vi "PDSS - Add Error Message.vi"(8 "error in (no error)":errorcluster, 9 "is warning? (False)":bool=TRUE, 10 "error code (0)":i32=5005, 11 "error message (\"\")":string) -> (0 "error out":errorcluster, 3 "Current Message":string)   [LabVIEW 2014]
doc: "Use this template to build a VI to use as a subVI."
panel:
  in  "show call chain? (False)":bool
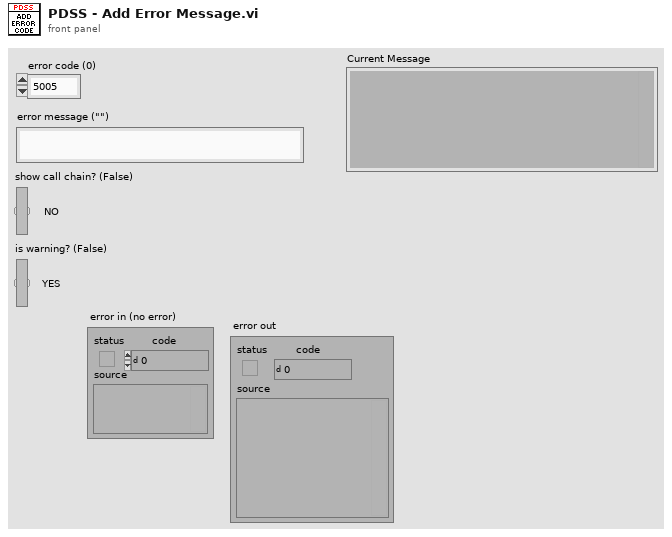
[diagram p1: front panel]
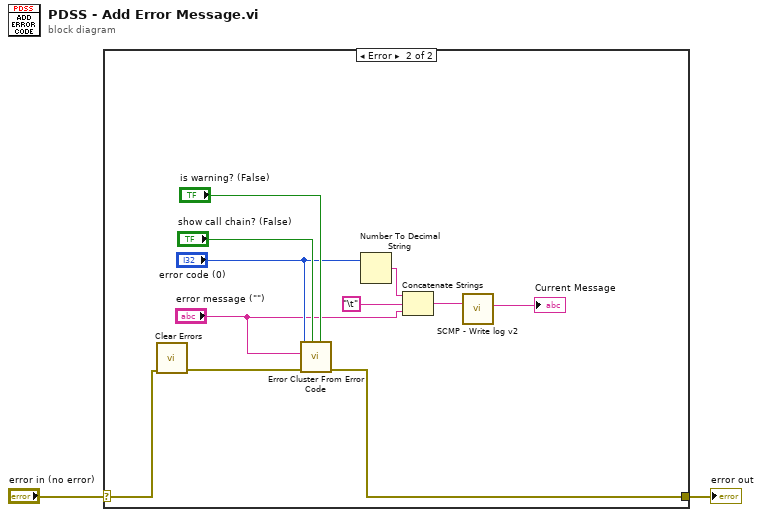
[diagram p0: block diagram]
diagram:
  n1 = case shown="Error" "error in (no error)" {
    selector: "error in (no error)" -> [w3 w14]
    tunnel: [w3 w12] -> w1
    frame No Error {
    }
    frame Error {
      n2 = call <vilib>:"Clear Errors.vi"("error in (no error)"=w14) -> ("error out"=w13:errorcluster)  [unwired: 5 in, 1 out]
      n3 = call <vilib>:"Error Cluster From Error Code.vi"("is warning? (False)"="is warning? (False)", "show call chain? (False)"="show call chain? (False)", "error in (no error)"=w13, "error message (\"\")"="error message (\"\")", "error code (0)"="error code (0)") -> ("error out"=w12:errorcluster)  [unwired: 4 in]
      n4 = Number To Decimal String(number="error code (0)") -> (decimal integer string=w8:string)  [unwired: 1 in]
      n5 = Concatenate Strings(w8, "\t", "error message (\"\")") -> (w5:string)
      n6 = call "SCMP - Write log v2.vi"("data"=w5) -> ("Last Log Entry"=→"Current Message":string)  [unwired: 8 in, 2 out]
    }
  }
  "error out" <- w1
